vi "Log Data.vi"(8 "error in (no error)":errorcluster, 10 "Data Queue":T1, 11 "Logging Configuration":T2) -> (0 "error out":errorcluster)   [LabVIEW 2018, in "Logging.lvlib"]
doc: "This VI uses the TDMS Write function to write data to a TDMS file."
uses:
  Logging.lvlib
  Logging Configuration.ctl
  Controls/Data Queue.ctl
  library/Datalogger LLB/Data Record Control.ctl
  library/Datalogger LLB/Datalogger.lvclass
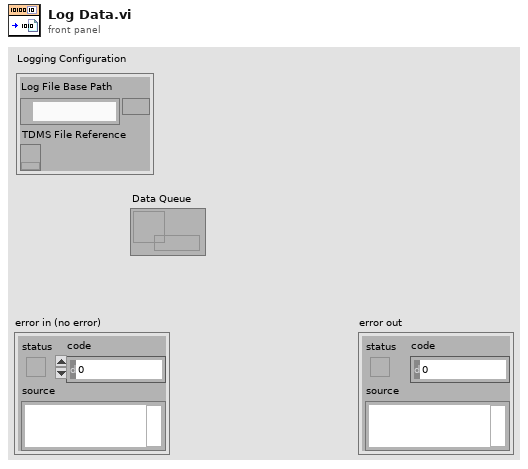
[diagram p1: front panel]
types:
  T1 = typedef "Data Queue.ctl" = refnum<queue>
  T2 = typedef "Logging.lvlib/Logging Configuration.ctl" = cluster{"Log File Base Path":path, "TDMS File Reference":refnum<k34>}
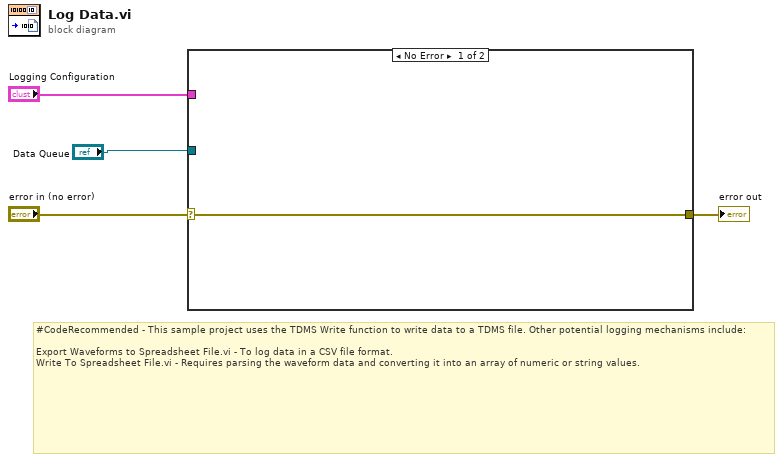
[diagram p0: block diagram]
diagram:
  # "#CodeRecommended - This sample project uses the TDMS Write function to write data to a TDMS file. Other potential logging mechanisms include:\n\nExport Waveforms to Spreadsheet File.vi - To log data in a CSV file format.\nWrite To Spreadsheet File.vi - Requires parsing the waveform data and converting it into an array of numeric or string values."
  n1 = case shown="No Error" "error in (no error)" {
    selector: "error in (no error)" -> [w5 w6]
    tunnel: "Logging Configuration" -> [_ _]
    tunnel: "Data Queue" -> [_ _]
    tunnel: [w5 w6] -> w3
    frame No Error {
    }
    frame Error {
    }
  }
  "error out" <- w3
